vi "Amplitude9225-7_FPGA.vi"(4 "dBin":fxp<+/-,36,0>, 5 "a":fxp<+,36,0>) -> (1 "Amplitude [p.u.]":fxp<+,36,0>)   [LabVIEW 2021]
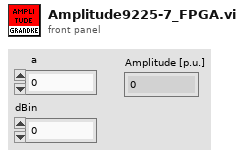
[diagram p1: front panel]
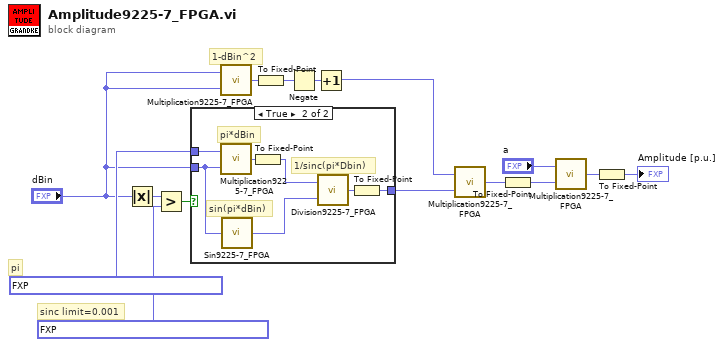
[diagram p0: block diagram]
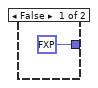
[diagram p2: hidden frame]
diagram:
  # "sinc limit=0.001"
  # "pi"
  # "1-dBin^2"
  n1 = Absolute Value(x="dBin") -> (abs(x)=w14:fxp<+,36,0>)
  n2 = Greater?(x=w14, y=fxp<+/-,36,0> 0.0010000000038417056) -> (0:w12:bool)
  n3 = case shown="True" w12 {
    tunnel: fxp<+,36,2> 3.1415926535846666 ("x") -> [_ w21]
    tunnel: [fxp<+/-,36,2> 1.0 ("x/y") w22] -> w10
    tunnel: "dBin" -> [_ w17]
    frame False {
    }
    frame True {
      # "1/sinc(pi*Dbin)"
      # "pi*dBin"
      # "sin(pi*dBin)"
      n4 = call "Multiplication9225-7_FPGA.vi"("y <+/-44,8>"=w17, "x <+/-47,6>"=w21) -> ("x*y <+/-49,13>"=w20:fxp<+/-,49,13>)
      n5 = call "Sin9225-7_FPGA.vi"("x [pi]"=w17) -> ("sin(x)"=w18:fxp<+/-,36,2>)
      n6 = To Fixed-Point(number=w20) -> (fixed-point=w19:fxp<+/-,36,2>)  [unwired: 1 in]
      n7 = call "Division9225-7_FPGA.vi"("y <+/-49,13>"=w18, "x <+/-40,4>"=w19) -> ("x/y <+/-38,4>"=w23:fxp<+/-,48,14>)
      n8 = To Fixed-Point(number=w23) -> (fixed-point=w22:fxp<+/-,36,2>)  [unwired: 1 in]
    }
  }
  n9 = call "Multiplication9225-7_FPGA.vi"("y <+/-44,8>"="dBin", "x <+/-47,6>"="dBin") -> ("x*y <+/-49,13>"=w4:fxp<+/-,49,13>)
  n10 = To Fixed-Point(number=w4) -> (fixed-point=w3:fxp<+,36,0>)  [unwired: 1 in]
  n11 = Negate(x=w3) -> (-x=w15:fxp<+/-,36,0>)
  n12 = Increment(x=w15) -> (x+1=w11:fxp<+,36,0>)
  n13 = call "Multiplication9225-7_FPGA.vi"("y <+/-44,8>"=w10, "x <+/-47,6>"=w11) -> ("x*y <+/-49,13>"=w9:fxp<+/-,49,13>)
  n14 = To Fixed-Point(number=w9) -> (fixed-point=w2:fxp<+,36,1>)  [unwired: 1 in]
  n15 = call "Multiplication9225-7_FPGA.vi"("y <+/-44,8>"=w2, "x <+/-47,6>"="a") -> ("x*y <+/-49,13>"=w7:fxp<+/-,49,13>)
  n16 = To Fixed-Point(number=w7) -> (fixed-point=→"Amplitude [p.u.]":fxp<+,36,0>)  [unwired: 1 in]
